vi "Set Definition Files.vi"(7 "application reference":refnum<vi>, 8 "error in (no error)":errorcluster, 10 "Channel Types":T1[](array[typedef]), 11 "owning references":T2) -> (0 "error out":errorcluster, 3 "owning references":T2)   [LabVIEW 2014, in "control module data interface generator.lvlib"]
uses:
  control module data interface generator.lvlib
  Controls/owning references.ctl
  <vilib>/NI/Tag Bus Module Framework/channel/channel classification.ctl
  <vilib>/Utility/traverseref.llb/TRef TravTarget.ctl
  <vilib>/Utility/traverseref.llb/VI Scripting - Traverse.lvlib
  <vilib>/NI/Tag Bus Module Framework/channel/TBM channel.lvclass
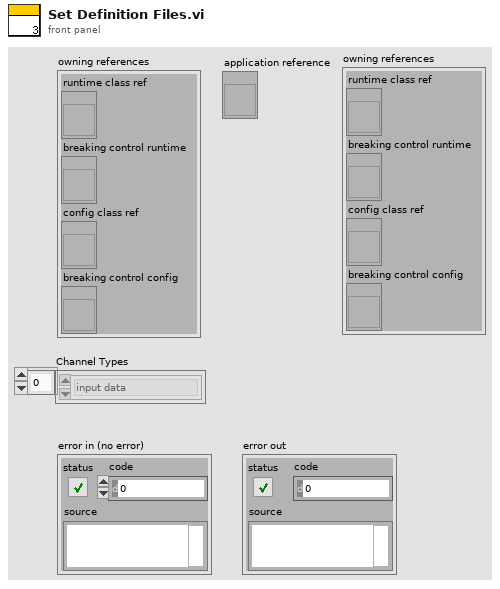
[diagram p1: front panel]
types:
  T1 = typedef "TBM channel.lvclass/channel classification.ctl" = enum16{"input data", "output data", "processing parameter", "processing result"}
  T2 = typedef "owning references.ctl" = cluster{"runtime class ref":refnum<vi>, "breaking control runtime":refnum<vi>, "config class ref":refnum<vi>, "breaking control config":refnum<vi>}
  T3 = typedef "TRef TravTarget.ctl" = enum16{"FP", "BD", "Other"}
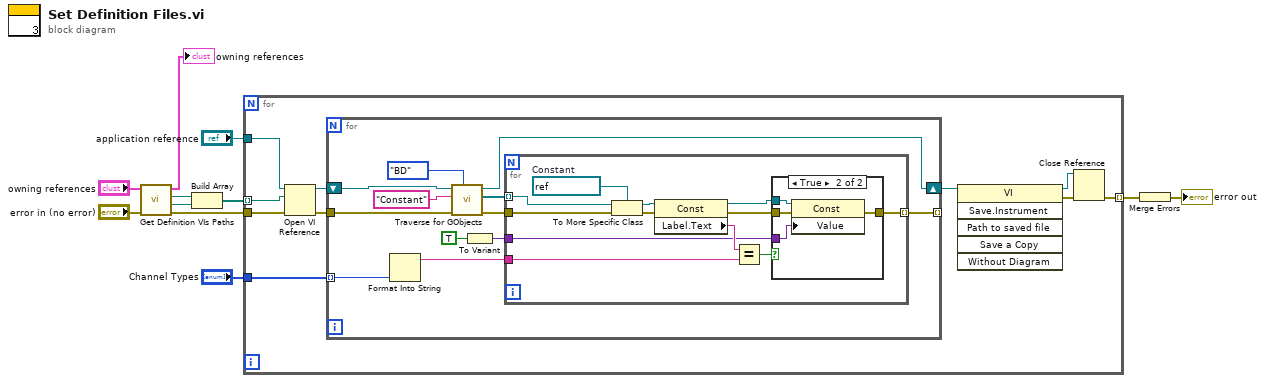
[diagram p0: block diagram]
diagram:
  n1 = call "Get Definition VIs Paths.vi"("error in (no error)"="error in (no error)", "owning references"="owning references") -> ("error out"=w3:errorcluster, "Get Index Definition"=w6:path, "Get Data Definition"=w7:path, "owning references 2"=→"owning references":T2)  [unwired: 6 in]
  n2 = Build Array(w7, w6) -> (w5:path[])
  n3 = for {
    tunnel: "Channel Types" -> [w21]
    tunnel: w5 -> [w20] mode=indexing
    tunnel: "application reference" -> [w19]
    tunnel: w3 -> [w18]
    tunnel: [w16] -> w2 mode=indexing
    n4 = Open VI Reference(application reference (local)=w19, vi path=w20, error in (no error)=w18) -> (vi reference=w15:refnum<vi>, error out=w13:errorcluster)  [unwired: 3 in]
    n5 = for {
      tunnel: w21 -> [w33] mode=indexing
      shift-right: [w27] -> w14
      shift-left: w15 -> [w30]
      tunnel: w13 -> [w25]
      tunnel: [w23] -> _ mode=indexing
      n6 = Format Into String(w33) -> (resulting string=w22:string)  [unwired: 3 in, 1 out]
      n7 = call <vilib>:"Traverse for GObjects.vi"("Traverse Target"=TRef_TravTarget."BD", "error in (no error)"=w25, "Class Name"="Constant", "VI Refnum"=w30) -> ("error out"=w24:errorcluster, "References"=w26:refnum<vi>[], "dup VI Refnum"=w27:refnum<vi>)  [unwired: 4 in, 1 out]
      n8 = To Variant(anything=TRUE) -> (Variant=w31:variant)
      n9 = for {
        tunnel: w31 -> [w34]
        tunnel: w26 -> [w45] mode=indexing
        tunnel: w24 -> [w43]
        tunnel: [w40] -> w23 mode=indexing
        tunnel: w22 -> [w36]
        w44 = refnum<vi> refnum  # Constant
        n10 = To More Specific Class(target class=w44, reference=w45, error in=w43) -> (specific class reference=w39:refnum<vi>, error out=w42:errorcluster)
        n11 = property class="Const"(reference=w39, error in=w42) -> (reference out=w38:refnum<vi>, error out=w41:errorcluster, "Label.Text"=w37:string)
        n12 = Equal?(x=w37, y=w36) -> (x = y?=w35:bool)
        n13 = case shown="True" w35 {
          tunnel: w41 -> [w46 w50]
          tunnel: [w46 w49] -> w40
          tunnel: w38 -> [_ w48]
          tunnel: w34 -> [_ w47]
          frame False {
          }
          frame True {
            n14 = property class="Const"(reference=w48, error in=w50, "Value"=w47) -> (error out=w49:errorcluster)  [unwired: 1 out]
          }
        }
      }
    }
    n15 = invoke class="VI" method="Save.Instrument"(reference=w14) -> (reference out=w12:refnum<vi>, error out=w17:errorcluster)  [unwired: 5 in, 4 out]
    n16 = Close Reference(reference=w12, error in (no error)=w17) -> (error out=w16:errorcluster)
  }
  n17 = Merge Errors(w2) -> (→"error out":errorcluster)
